vi "Remove_Apple_Hidden_Files.vi"(1 "Files In":string[](array[string])) -> (0 "Files Out":string[](array[string]))   [LabVIEW 2012]
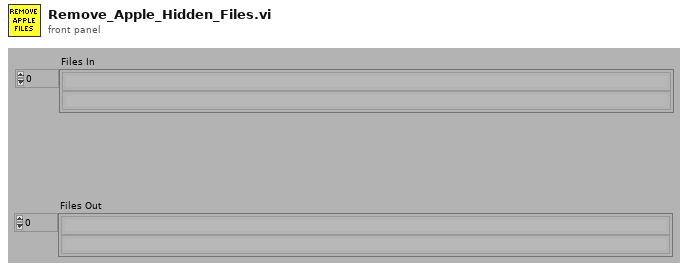
[diagram p1: front panel]
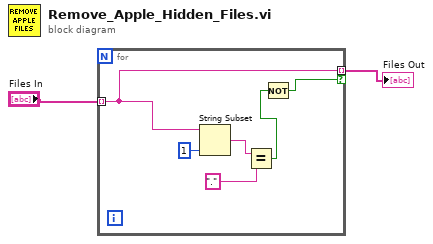
[diagram p0: block diagram]
diagram:
  n1 = for {
    tunnel: "Files In" -> [w3] mode=indexing
    tunnel: [w3] -> w2 mode=indexing if=w8
    n2 = String Subset(string=w3, length (rest)=1 ("length (rest)")) -> (substring=w6:string)  [unwired: 1 in]
    n3 = Equal?(x=w6, y=".") -> (x = y?=w4:bool)
    n4 = Not(x=w4) -> (.not. x?=w8:bool)
  }
  "Files Out" <- w2
